vi "RichToFlatnixnet_grpc_ReadSignalSinglePointResponse.vi"(5 "OutputClusterType":T1, 11 "InputCluster":T2) -> (3 "OutputCluster":T1)   [LabVIEW 2025, in "grpc-xnet_client.lvlib"]
uses:
  nixnet_grpc_ReadSignalSinglePointResponse.ctl
  nixnet_grpc_ReadSignalSinglePointResponse_Flat.ctl
  grpc-xnet_client.lvlib
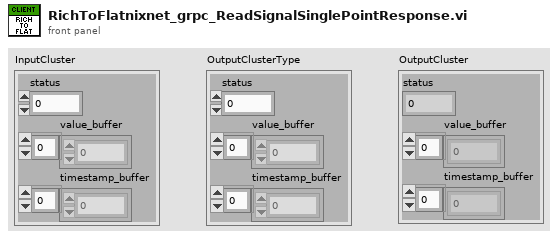
[diagram p1: front panel]
types:
  T1 = typedef "grpc-xnet_client.lvlib/nixnet_grpc_ReadSignalSinglePointResponse_Flat.ctl" = cluster{"status":i32, "value_buffer":dbl[], "timestamp_buffer":u64[]}
  T2 = typedef "grpc-xnet_client.lvlib/nixnet_grpc_ReadSignalSinglePointResponse.ctl" = cluster{"status":i32, "value_buffer":dbl[], "timestamp_buffer":u64[]}
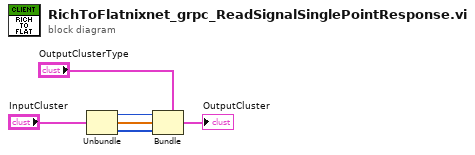
[diagram p0: block diagram]
diagram:
  n1 = Unbundle "Unbundle"("InputCluster") -> ("status"=w3:i32, "value_buffer"=w2:dbl[], "timestamp_buffer"=w1:u64[])
  n2 = Bundle "Bundle"(cluster="OutputClusterType", "status"=w3, "value_buffer"=w2, "timestamp_buffer"=w1) -> (→"OutputCluster":T1)
